vi "Read Element of Cameras.vi"(8 "error in (no error)":errorcluster, 10 "index":i32, 11 "Gantry Class in":refnum<class "Gantry Class.lvclass">) -> (0 "error out":errorcluster, 2 "Camera":cluster{"Name":string, "IMAQ Session":T1}, 3 "Gantry Class out":refnum<class "Gantry Class.lvclass">)   [LabVIEW 2011, in "Gantry Class.lvclass"]
uses:
  Gantry Class.lvclass
  <vilib>/userdefined/High Color/IMAQdx.ctl
  Gantry Class.lvclass/Gantry Class.ctl
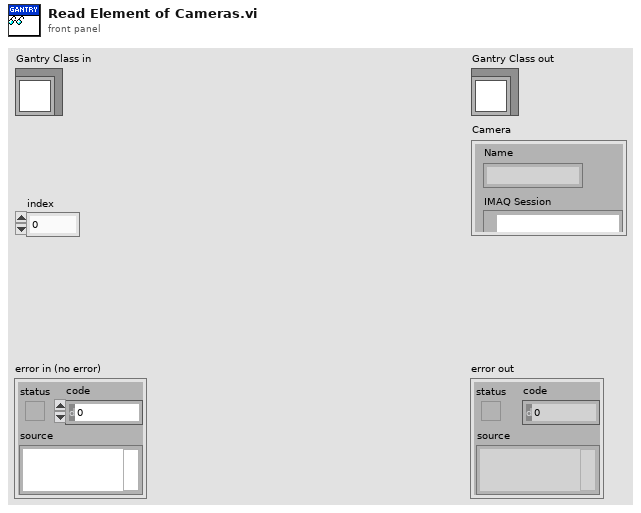
[diagram p1: front panel]
types:
  T1 = typedef "IMAQdx.ctl" = refnum<k21>
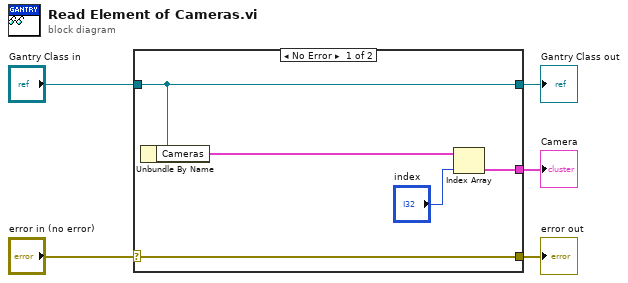
[diagram p0: block diagram]
diagram:
  n1 = case shown="No Error" "error in (no error)" {
    selector: "error in (no error)" -> [w10 w11]
    tunnel: [w10 w11] -> w4
    tunnel: [w9 w12] -> w2
    tunnel: "Gantry Class in" -> [w9 w12]
    tunnel: [w6 _] -> w1
    frame No Error {
      n2 = Unbundle By Name(w9) -> ("Cameras"=w8:cluster{"Name":string, "IMAQ Session":T1}[])
      n3 = Index Array(array=w8, index="index") -> (element=w6:cluster{"Name":string, "IMAQ Session":T1})
    }
    frame Error {
    }
  }
  "error out" <- w4
  "Gantry Class out" <- w2
  "Camera" <- w1
